vi "Update.vi"(8 "error in (no error)":errorcluster, 10 "Model in":refnum<class "Model.lvclass">, 11 "Perform Open Loop Scan State in":refnum<class "Perform Scan State.lvclass">) -> (0 "error out":errorcluster, 2 "Model out":refnum<class "Model.lvclass">, 3 "Perform Open Loop Scan State out":refnum<class "Perform Scan State.lvclass">)   [LabVIEW 2015, in "Perform Scan State.lvclass"]
uses:
  Perform Scan State.lvclass
  Model/Model/Model.lvclass
  Typedefs/StateTypes.ctl
  Typedefs/FAMT Typedefs.lvlib
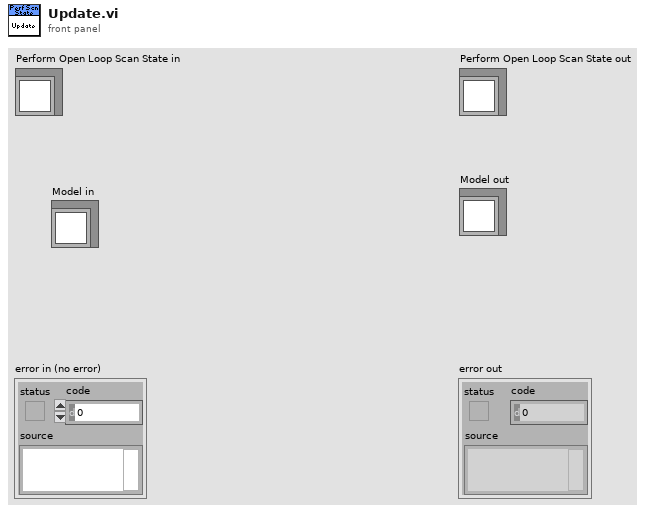
[diagram p1: front panel]
types:
  T1 = typedef "FAMT Typedefs.lvlib/StateTypes.ctl" = enum16{"Offline State", "Fault State", "Standby State", "Disabled State", "Enabled State", "Wait For User Input State", "Perform Scan State"}
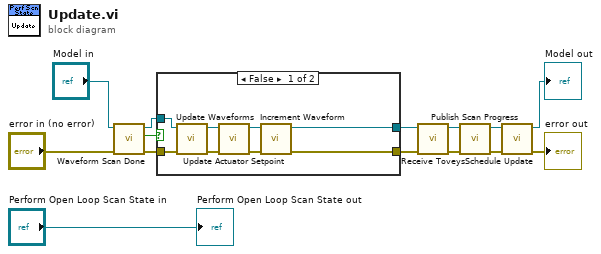
[diagram p0: block diagram]
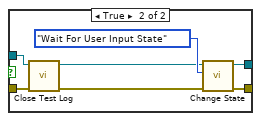
[diagram p2: hidden frame]
diagram:
  n1 = call "Waveform Scan Done.vi"("error in (no error)"="error in (no error)", "Model in"="Model in") -> ("error out"=w8:errorcluster, "Done"=w11:bool, "Model out"=w10:refnum<class "Model.lvclass">)  [unwired: 7 in]
  n2 = case shown="False" w11 {
    tunnel: w10 -> [w21 w26]
    tunnel: [w16 w23] -> w1
    tunnel: [w15 w24] -> w2
    tunnel: w8 -> [w20 w25]
    frame False {
      n3 = call "Update Waveforms.vi"("error in (no error)"=w20, "Model in"=w21) -> ("error out"=w19:errorcluster, "Model out"=w22:refnum<class "Model.lvclass">)  [unwired: 8 in]
      n4 = call "Update Actuator Setpoint.vi"("error in (no error)"=w19, "Model in"=w22) -> ("error out"=w17:errorcluster, "Model out"=w18:refnum<class "Model.lvclass">)  [unwired: 8 in]
      n5 = call "Increment Waveform.vi"("error in (no error)"=w17, "Model in"=w18) -> ("error out"=w16:errorcluster, "Model out"=w15:refnum<class "Model.lvclass">)  [unwired: 8 in]
    }
    frame True {
      n6 = call "Close Test Log.vi"("error in (no error)"=w25, "Model in"=w26) -> ("error out"=w27:errorcluster, "Model out"=w28:refnum<class "Model.lvclass">)  [unwired: 8 in]
      n7 = call "Change State.vi"("error in (no error)"=w27, "State Types"=StateTypes."Wait For User Input State" ("State:"), "Model in"=w28) -> ("error out"=w23:errorcluster, "Model out"=w24:refnum<class "Model.lvclass">)  [unwired: 7 in]
    }
  }
  n8 = call "Receive Toveys.vi"("error in (no error)"=w1, "Model in"=w2) -> ("error out"=w4:errorcluster, "Model out"=w3:refnum<class "Model.lvclass">)  [unwired: 8 in]
  n9 = call "Publish Scan Progress.vi"("error in (no error)"=w4, "Model in"=w3) -> ("error out"=w7:errorcluster, "Model out"=w12:refnum<class "Model.lvclass">)  [unwired: 8 in]
  n10 = call "Schedule Update.vi"("error in (no error)"=w7, "Model in"=w12) -> ("error out"=→"error out":errorcluster, "Model out"=→"Model out":refnum<class "Model.lvclass">)  [unwired: 8 in]
  "Perform Open Loop Scan State out" <- "Perform Open Loop Scan State in"
